vi "INDEX-generator-main.vi"(6 "header":string, 8 "error in":errorcluster, 9 "report file destination":path=path "/Macintosh HD/Users/oddoa/Work/LabVIEW/Vi-Documentation/generated", 10 "tasks":T1[](array[typedef])=[{"State machine"=enum."add-red-box-header", "HTML before"="", "HTML after"=""}, {"State machine"=enum."Add VI description", "HTML before"="<h1>My Main Tool description</h1>\n<h2>Where it all began</h2> \n<br>", "HTML after"=""}, {"State machine"=enum."Add front panel", "HTML before"="<h1>Front Panel visible view</h1>\njust some text about the VI <br>", "HTML after"="<br>Picture text if one desires"}, {"State machine"=enum."Add Block Diagram", "HTML before"="<h1> Code</h1>\n<br>", "HTML after"=""}, {"State machine"=enum."Add VI hiearchy", "HTML before"="<h1>VI hiearchy</h1>\n<br>", "HTML after"=""}], 11 "VI paths":path[](array[path])) -> (0 "error out":errorcluster)   [LabVIEW 2014]
uses:
  controls/state program.ctl
  controls/state-machine.ctl
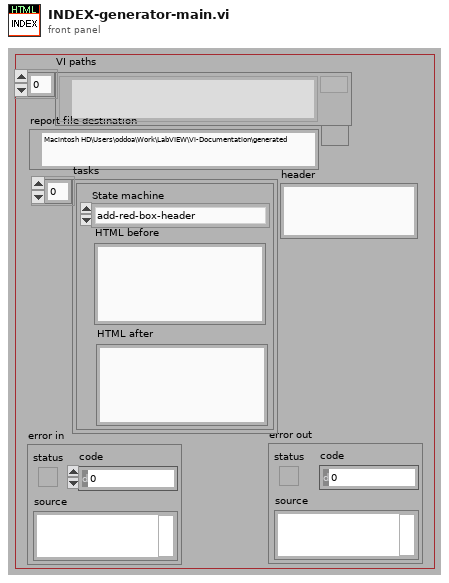
[diagram p1: front panel]
types:
  T1 = typedef "state program.ctl" = cluster{"State machine":T2, "HTML before":string, "HTML after":string}
  T2 = typedef "state-machine.ctl" = enum16{"add carridge return", "init", "Read-inputs", "edit generated file", "end", "Add front panel", "Add Block Diagram", "Add VI icon", "Add VI description", "Add VI hiearchy", "Add list of sub vis", "add custom html", "open report in browser", "Save report to file", "dispose report", "Add header text", "Create style .css", "add-red-box-header", "Delete Temp Files", "Remove-path-element", "add-revision-history", "add-icon-image-only"}
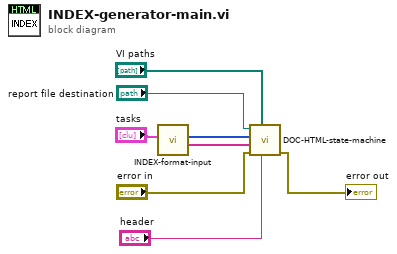
[diagram p0: block diagram]
diagram:
  n1 = call "INDEX-format-input.vi"("tasks"="tasks") -> ("HTML"=w3:string[], "states"=w4:T2[])  [unwired: 9 out]
  n2 = call "DOC-HTML-state-machine.vi"("header"="header", "VI paths"="VI paths", "error in"="error in", "HTML"=w3, "states"=w4, "report file destination"="report file destination") -> ("error out"=→"error out":errorcluster)  [unwired: 3 in, 2 out]
